vi "IniPath.vi"() -> (3 "INI Path":path)   [LabVIEW 2014]
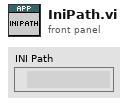
[diagram p1: front panel]
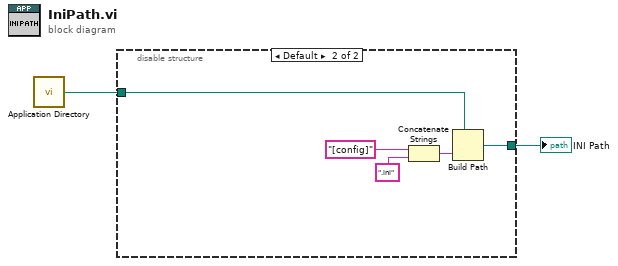
[diagram p0: block diagram]
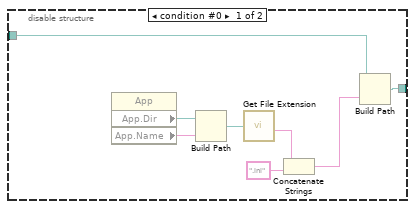
[diagram p2: hidden frame]
diagram:
  n1 = call <vilib>:"Application Directory.vi"() -> ("Application Directory"=w1:path)
  n2 = disable-structure shown="Default" {
    disable-tunnel: [w10 w12] -> w2
    disable-tunnel: w1 -> [w9 w11]
    frame condition #0 {
      n3 = property class="App"() -> ("App.Dir"=w7:path, "App.Name"=w6:string)  [unwired: 2 in, 2 out]
      n4 = Build Path(base path=w7, name or relative path=w6) -> (appended path=w5:path)
      n5 = call <vilib>:"Get File Extension.vi"("file"=w5) -> ("filename without extension"=w4:string)  [unwired: 7 in, 3 out]
      n6 = Concatenate Strings(w4, ".ini" ("Application:Name")) -> (w3:string)
      n7 = Build Path(base path=w9, name or relative path=w3) -> (appended path=w10:path)
    }
    frame condition #1 (active) {
      n8 = Concatenate Strings("[config]" ("string"), ".ini" ("Application:Name")) -> (w14:string)
      n9 = Build Path(base path=w11, name or relative path=w14) -> (appended path=w12:path)
    }
  }
  "INI Path" <- w2
